vi "ZCAN_InitCAN(USBCANFD).vi"(0 "device_hande":u32, 5 "can_index":u32, 7 "ZCAN_InitCAN_Setting_USBCANFD":T1={"abitbaud"=500000, "dbitbaud"=500000, "CustomBaud"=FALSE, "CustomBd"="", "Mode"=0, "Standard"=0} {"Standard" items=["CANFD ISO", "CANFD BOSCH"]; "dbitbaud" items=["5Mbps"=5000000, "4Mbps"=4000000, "2Mbps"=2000000, "1Mbps"=1000000, "800kbps"=800000, "500kbps"=500000, "250kbps"=250000, "125kbps"=125000, "100kbps"=100000]; "abitbaud" items=["1Mbps"=1000000, "800kbps"=800000, "500kbps"=500000, "250kbps"=250000, "125kbps"=125000, "100kbps"=100000, "50kbps"=50000]; "Mode" items=["正常", "只听"]}, 11 "error in (no error)":errorcluster caption="错误输入（无错误）") -> (8 "can_index_handle":u32, 15 "error out":errorcluster caption="错误输出")   [LabVIEW 2011, in "zlgcan.lvlib"]
doc: "设置CAN卡波特率，工作模式等。\n\n适用的设备：USBCANFD-100U、USBCANFD-200U、USBCANFD-MINI。"
uses:
  zlgcan.lvlib
  bin/ControlCANFD.dll
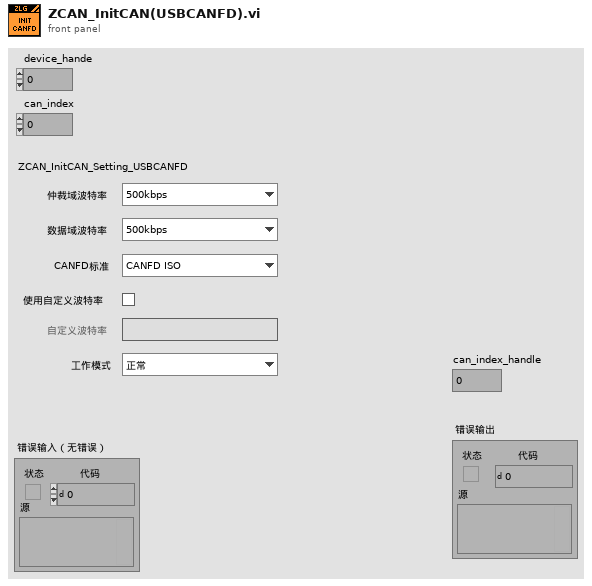
[diagram p1: front panel]
types:
  T1 = cluster{"abitbaud":u32, "dbitbaud":u32, "CustomBaud":bool, "CustomBd":string, "Mode":u8, "Standard":u32}
  T2 = cluster{"can_type":u32, "can_type":u32, "can_type":u32, "can_type":u32, "can_type":u32, "can_type":u32, u8, "Mode":u8, "pad":u16, "reserved":u32}
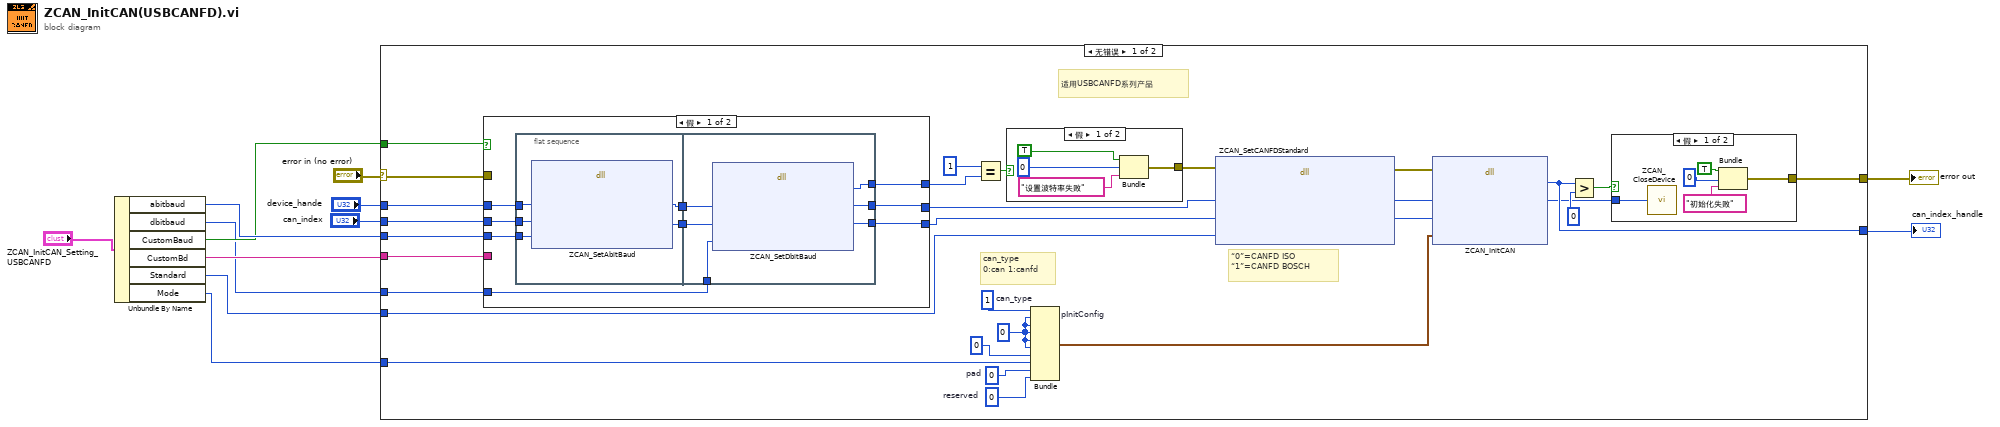
[diagram p0: block diagram]
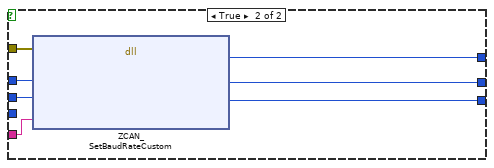
[diagram p4: hidden frame]
diagram:
  n1 = Unbundle By Name("ZCAN_InitCAN_Setting_USBCANFD") -> ("abitbaud"=w6:u32, "dbitbaud"=w2:u32, "CustomBaud"=w5:bool, "CustomBd"=w4:string, "Standard"=w1:u32, "Mode"=w3:u8)
  n2 = case shown="无错误" "error in (no error)" {
    selector: "error in (no error)" -> [w36 w78]
    tunnel: [w35 w78] -> w11
    tunnel: w5 -> [w41 _]
    tunnel: "device_hande" -> [w40 _]
    tunnel: "can_index" -> [w39 _]
    tunnel: w6 -> [w38 _]
    tunnel: w4 -> [w37 _]
    tunnel: w3 -> [w21 _]
    tunnel: [w34 _] -> w8
    tunnel: w2 -> [w15 _]
    tunnel: w1 -> [w13 _]
    frame No Error {
      w22 = u32 0  # reserved
      w23 = u16 0  # pad
      w20 = u32 0 ("can_type")
      w24 = u32 1  # can_type
      # "can_type\n0:can 1:canfd"
      # "“0”=CANFD ISO \n“1”=CANFD BOSCH"
      # "适用USBCANFD系列产品"
      n3 = case shown="假" w41 {
        tunnel: [w52 w77] -> w27
        tunnel: [w51 w76] -> w26
        tunnel: [w53 w75] -> w32
        tunnel: w40 -> [w59 w73]
        tunnel: w39 -> [w58 w72]
        tunnel: w38 -> [w57 _]
        tunnel: w37 -> [_ w74]
        tunnel: w36 -> [_ w71]
        tunnel: w15 -> [w54 _]
        frame False {
          n4 = flat-sequence {
            tunnel: w59 -> [w62]
            tunnel: w58 -> [w61]
            tunnel: w57 -> [w60]
            tunnel: [w64] -> w56
            tunnel: [w63] -> w55
            tunnel: w56 -> [w70]
            tunnel: w55 -> [w69]
            tunnel: w54 -> [w68]
            tunnel: [w67] -> w53
            tunnel: [w66] -> w52
            tunnel: [w65] -> w51
            frame #0 {
              n5 = dll-call lib="C:/Users/ttc52/Desktop/DHC FD LV2018/LABIVIEW2011 CANFD Tool_V1.2.4_x86_20250428/bin/ControlCANFD.dll" fn="ZCAN_SetAbitBaud" label="设置仲裁域波特率"("device_hande"=w62, "can_index"=w61, "abitbaud"=w60) -> ("device_hande"=w64:u32, "can_index"=w63:u32)  [unwired: 5 in, 2 out]
            }
            frame #1 {
              n6 = dll-call lib="C:/Users/ttc52/Desktop/DHC FD LV2018/LABIVIEW2011 CANFD Tool_V1.2.4_x86_20250428/bin/ControlCANFD.dll" fn="ZCAN_SetDbitBaud" label="设置数据域波特率"("device_hande"=w70, "can_index"=w69, "dbitbaud"=w68) -> ("return"=w67:u32, "device_hande"=w66:u32, "can_index"=w65:u32)  [unwired: 4 in, 2 out]
            }
          }
        }
        frame True {
          n7 = dll-call lib="C:/Users/ttc52/Desktop/DHC FD LV2018/LABIVIEW2011 CANFD Tool_V1.2.4_x86_20250428/bin/ControlCANFD.dll" fn="ZCAN_SetBaudRateCustom"(error in=w71, "device_handle"=w73, "can_index"=w72, "RateCustom"=w74) -> ("return"=w75:u32, "device_handle"=w77:u32, "can_index"=w76:u32)  [unwired: 3 in, 2 out]
        }
      }
      n8 = Equal?(x=1, y=w32) -> (x = y?=w31:bool)
      n9 = case shown="假" w31 {
        tunnel: [w47 _] -> w28
        frame False {
          n10 = Bundle("status"=TRUE, "code"=0, "消息"="设置波特率失败") -> (w47:cluster{"status":bool, "code":i32, "消息":string})  [unwired: 1 in]
        }
        frame True {
        }
      }
      n11 = Bundle "pInitConfig"("can_type"=w24, "can_type"=w20, "can_type"=w20, "can_type"=w20, "can_type"=w20, "can_type"=w20, u8 0, "Mode"=w21, "pad"=w23, "reserved"=w22) -> (w18:T2)  [unwired: 1 in]
      n12 = dll-call lib="C:/Users/ttc52/Desktop/DHC FD LV2018/LABIVIEW2011 CANFD Tool_V1.2.4_x86_20250428/bin/ControlCANFD.dll" fn="ZCAN_SetCANFDStandard" ("ZCAN_InitCAN")(error in=w28, "device_handle"=w27, "can_index"=w26, "canfd_standard"=w13) -> (error out=w25:errorcluster, "device_handle"=w17:u32, "can_index"=w16:i32)  [unwired: 4 in, 1 out]
      n13 = dll-call lib="C:/Users/ttc52/Desktop/DHC FD LV2018/LABIVIEW2011 CANFD Tool_V1.2.4_x86_20250428/bin/ControlCANFD.dll" fn="ZCAN_InitCAN"(error in=w25, "device_handle"=w17, "can_index"=w16, "pInitConfig"=w18) -> ("can_handle"=w34:u32, "device_handle"=w14:u32)  [unwired: 4 in, 2 out]
      n14 = Greater?(x=w34, y=0) -> (0:w29:bool)
      n15 = case shown="假" w29 {
        tunnel: [w43 _] -> w35
        tunnel: w14 -> [w42 _]
        frame False {
          n16 = call "ZCAN_CloseDevice.vi"("device_handle"=w42) -> ()  [unwired: 9 in, 2 out]
          n17 = Bundle("status"=TRUE, "code"=0, "消息"="初始化失败") -> (w43:cluster{"status":bool, "code":i32, "消息":string})  [unwired: 1 in]
        }
        frame True {
        }
      }
    }
    frame Error {
    }
  }
  "error out" <- w11
  "can_index_handle" <- w8
